vi "Reset Buffer Size.vi"(4 "Error In":errorcluster, 7 "New Buffer Size":i32) -> (0 "Error Out":errorcluster)   [LabVIEW 2015, in "Ramp Signal Data Buffer.lvlib"]
uses:
  Ramp Signal Data Buffer.lvlib
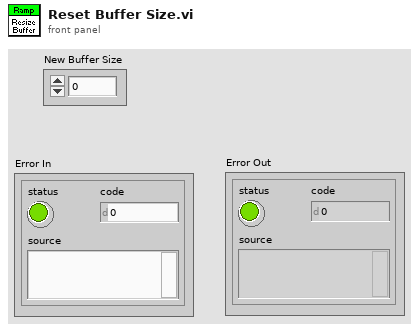
[diagram p1: front panel]
types:
  T1 = typedef "Ramp Signal Data Buffer.lvlib/buffer data typedef.ctl" = cluster{"Ramp Data":dbl[], "Counter":i32}
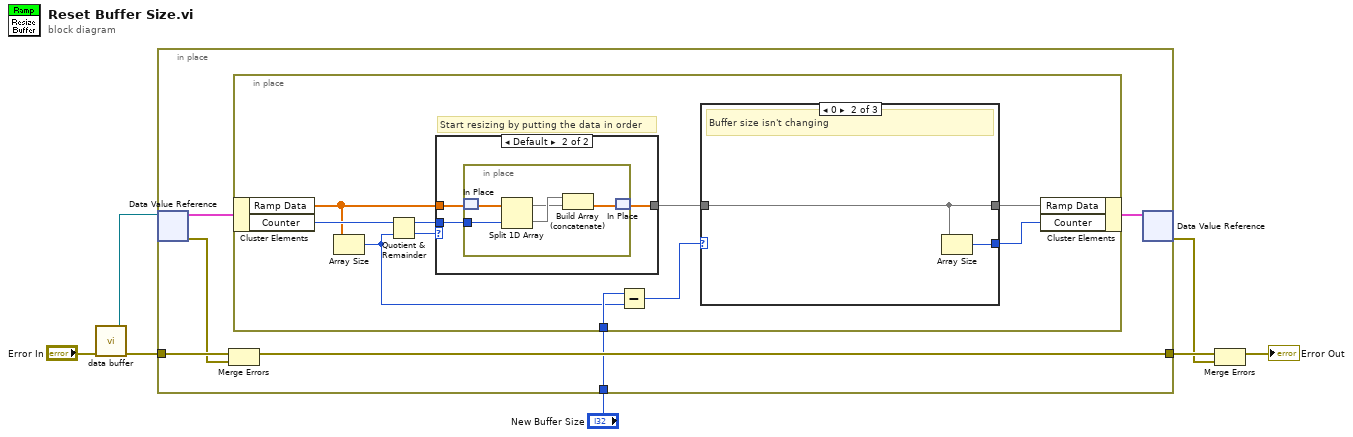
[diagram p0: block diagram]
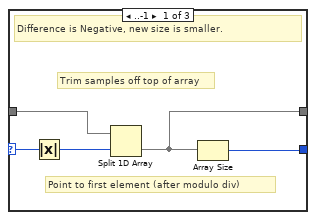
[diagram p2: hidden frame]
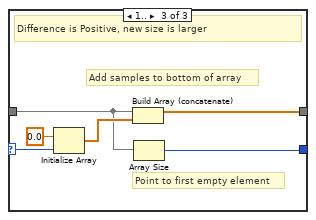
[diagram p3: hidden frame]
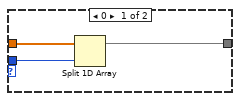
[diagram p4: hidden frame]
diagram:
  n1 = call "data buffer.vi"("Error In"="Error In") -> ("Error Out"=w5:errorcluster, "DVR"=w4:refnum<data-value>)  [unwired: 5 in]
  n2 = in-place {
    in-place-border: w5 -> [w13]
    in-place-border: [w12] -> w6
    in-place-border: "New Buffer Size" -> [w8]
    n3 = in-place-dvr #1(w4) -> (w10:T1, w11:errorcluster)
    n4 = Merge Errors(w13, w11) -> (w12:errorcluster)
    n5 = in-place {
      in-place-border: w8 -> [w15]
      # "Start resizing by putting the data in order"
      n6 = in-place-cluster #2(w10) -> ("Ramp Data"=w17:dbl[], "Counter"=w21:i32)
      n7 = Array Size(array=w17) -> (size(s)=w14:i32)
      n8 = Quotient & Remainder(x=w21, y=w14) -> (x-y*floor(x/y)=w22:i32, floor(x/y)=w23:i32)
      n9 = case shown="Default" w23 {
        tunnel: w17 -> [w39 w42]
        tunnel: [w37 w41] -> w20
        tunnel: w22 -> [w38 w40]
        frame 0 {
          n10 = Split 1D Array(array=w39, index=w38) -> (first subarray=w37:dbl[])  [unwired: 1 out]
        }
        frame Default {
          n11 = in-place {
            in-place-border: w40 -> [w47]
            n12 = in-place-match #3(w42) -> (w44:dbl[])
            n13 = Split 1D Array(array=w44, index=w47) -> (first subarray=w45:dbl[], second subarray=w46:dbl[])
            n14 = Build Array (concatenate)(w46, w45) -> (w43:dbl[])
            n15 = in-place-match #3(w43) -> (w41:dbl[])
          }
        }
      }
      n16 = Subtract(x=w15, y=w14) -> (x-y=w16:i32)
      n17 = case shown="0" w16 {
        selector: w16 -> [w28 _ w36]
        tunnel: w20 -> [w26 w30 w32]
        tunnel: [w24 w29 w31] -> w19
        tunnel: [w25 w30 w33] -> w18
        frame ..-1 {
          # "Point to first element (after modulo div)"
          # "Trim samples off top of array"
          # "Difference is Negative, new size is smaller."
          n18 = Absolute Value(x=w28) -> (abs(x)=w27:i32)
          n19 = Split 1D Array(array=w26, index=w27) -> (second subarray=w25:dbl[])  [unwired: 1 out]
          n20 = Array Size(array=w25) -> (size(s)=w24:i32)
        }
        frame 0 {
          # "Buffer size isn't changing"
          n21 = Array Size(array=w30) -> (size(s)=w29:i32)
        }
        frame 1.. {
          # "Point to first empty element"
          # "Add samples to bottom of array"
          # "Difference is Positive, new size is larger"
          n22 = Initialize Array(0.0 ("element"), w36) -> (w34:dbl[])
          n23 = Build Array (concatenate)(w32, w34) -> (w33:dbl[])
          n24 = Array Size(array=w32) -> (size(s)=w31:i32)
        }
      }
      n25 = in-place-cluster #2("Ramp Data"=w18, "Counter"=w19) -> (w9:T1)
    }
    n26 = in-place-dvr #1(w9) -> (w3:errorcluster)  [unwired: 1 out]
  }
  n27 = Merge Errors(w6, w3) -> (→"Error Out":errorcluster)
